vi "Concatenate State with Arguments.vi"(10 "Arguments":string, 11 "State":string) -> (3 "State With Arguements":string)   [LabVIEW 2017, in "CSM Shared.lvlib"]
doc: "### Concatenate State with Arguments.vi\n\n-- <b>Controls</b> --\n- <b>Arguments</b>:\n- <b>State</b>:\n\n-- <b>Indicators</b> --\n- <b>State with Arguments</b>:"
uses:
  CSM Shared.lvlib
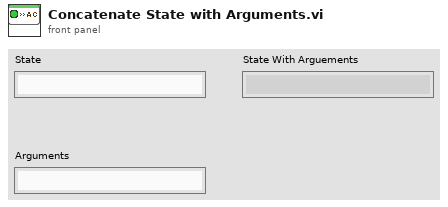
[diagram p1: front panel]
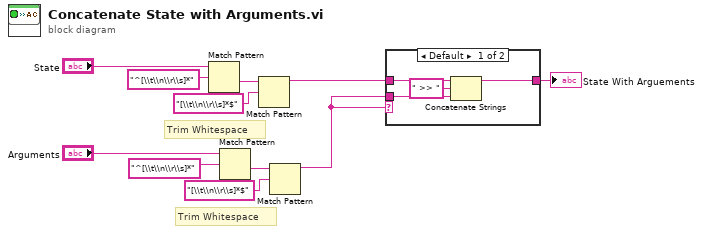
[diagram p0: block diagram]
diagram:
  # "Trim Whitespace"
  # "Trim Whitespace"
  n1 = Match Pattern(string="State", regular expression="^[\\t\\n\\r\\s]*") -> (after substring=w9:string)  [unwired: 1 in, 3 out]
  n2 = Match Pattern(string="Arguments", regular expression="^[\\t\\n\\r\\s]*") -> (after substring=w4:string)  [unwired: 1 in, 3 out]
  n3 = Match Pattern(string=w9, regular expression="[\\t\\n\\r\\s]*$") -> (before substring=w6:string)  [unwired: 1 in, 3 out]
  n4 = Match Pattern(string=w4, regular expression="[\\t\\n\\r\\s]*$") -> (before substring=w1:string)  [unwired: 1 in, 3 out]
  n5 = case "Is arguments empty? If so, then do not append arguments" shown="Default" w1 {
    tunnel: [w12 w16] -> w11
    tunnel: w6 -> [w15 w16]
    tunnel: w1 -> [w13 _]
    frame Default {
      n6 = Concatenate Strings(w15, " >> " ("string"), w13) -> (w12:string)
    }
    frame "" {
    }
  }
  "State With Arguements" <- w11
